vi "Convert 2D image to 2D array FPGA.vi"(11 "image data":T1) -> (3 "data":u16[][](array[numeric]))   [LabVIEW 2019]
uses:
  <vilib>/picture/picture.llb/imagedata.ctl
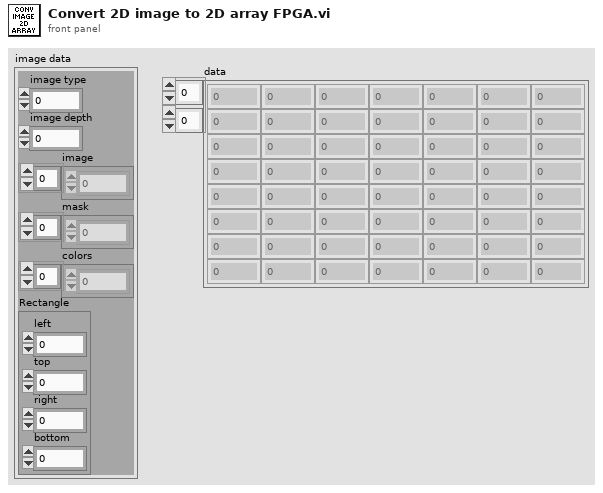
[diagram p1: front panel]
types:
  T1 = typedef "imagedata.ctl" = cluster{"image type":i32, "image depth":i32, "image":u8[], "mask":u8[], "colors":u32[], "Rectangle":cluster{"left":i16, "top":i16, "right":i16, "bottom":i16}}
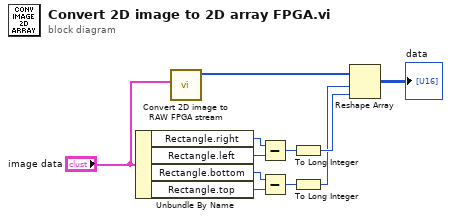
[diagram p0: block diagram]
diagram:
  n1 = Unbundle By Name("image data") -> ("Rectangle.right"=w2:i16, "Rectangle.left"=w3:i16, "Rectangle.bottom"=w4:i16, "Rectangle.top"=w5:i16)
  n2 = call "Convert 2D image to RAW FPGA stream.vi"("image data"="image data") -> ("data"=w11:u16[])  [unwired: 9 in, 1 out]
  n3 = Subtract(x=w2, y=w3) -> (x-y=w6:i16)
  n4 = Subtract(x=w4, y=w5) -> (x-y=w7:i16)
  n5 = To Long Integer(number=w6) -> (32bit integer=w10:i32)
  n6 = To Long Integer(number=w7) -> (32bit integer=w9:i32)
  n7 = Reshape Array(w11, w9, w10) -> (→"data":u16[][])
